vi "Configure Modulation (Phase).vi"(0 "VISA resource name":refnum<visa-resource-name>, 1 "Enable Phase Modulation (T: Enable)":bool=TRUE, 5 "Channel (0: Channel 1)":u16(ring) items=["Channel 1", "Channel 2"], 7 "PM Source (0: Internal)":u16(ring) items=["Internal", "External"], 9 "Modulation Waveform (0: Sine)":u16(ring) items=["Sine", "Square", "Triangle", "Ramp", "Down Ramp", "Noise", "User 1", "User 2", "User 3", "User 4", "Edit Memory"], 11 "error in (no error)":errorcluster, 12 "Modulation Frequency (100.00 Hz)":dbl=100.0 format="%#_6f", 13 "Peak Deviation (90 deg)":dbl=90.0 min=-180.0 max=180.0 format="%#.4f") -> (4 "VISA resource name out":refnum<visa-resource-name>, 15 "error out":errorcluster)   [LabVIEW 2013, in "Tektronix AFG 3000 Series.lvlib"]
doc: "Configures and enables phase modulation (PM). In PM, the phase of the carrier is varied by the peak deviation and the modulating waveform. \n\n<B>Note:</B>\n\nDefault measure for peak deviation is in degrees only. To change deviation unit to radians replace the DEG with RAD in the peak deviation command."
uses:
  Tektronix AFG 3000 Series.lvlib
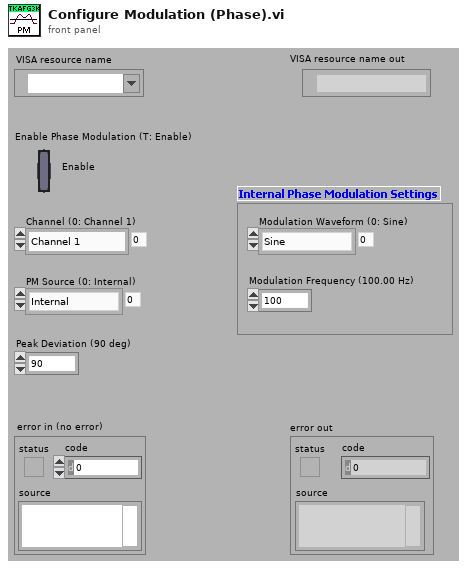
[diagram p1: front panel]
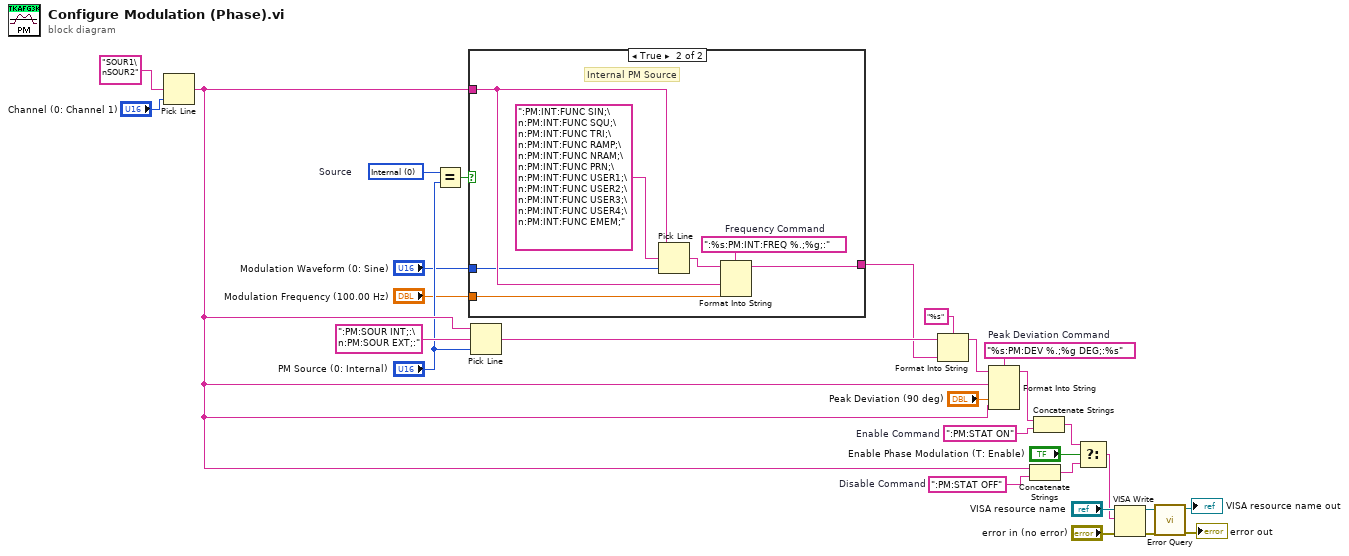
[diagram p0: block diagram]
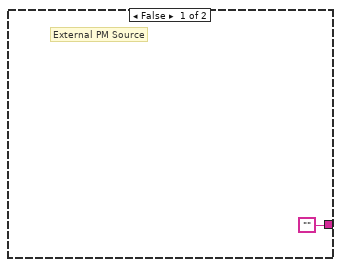
[diagram p2: hidden frame]
diagram:
  w20 = ":PM:STAT ON"  # Enable Command
  w22 = "%s:PM:DEV %.;%g DEG;:%s"  # Peak Deviation Command
  w9 = u16 0 items=["Internal", "External"]  # Source
  w17 = ":PM:STAT OFF"  # Disable Command
  n1 = Pick Line(multi-line string="SOUR1\nSOUR2" ("string (\"\")"), line index="Channel (0: Channel 1)") -> (output string=w11:string)  [unwired: 1 in]
  n2 = Equal?(x=w9, y="PM Source (0: Internal)") -> (x = y?=w8:bool)
  n3 = case shown="True" w8 {
    tunnel: ["" w33] -> w4
    tunnel: w11 -> [_ w32]
    tunnel: "Modulation Waveform (0: Sine)" -> [_ w31]
    tunnel: "Modulation Frequency (100.00 Hz)" -> [_ w30]
    frame False {
      # "External PM Source"
    }
    frame True {
      w34 = ":%s:PM:INT:FREQ %.;%g;:"  # Frequency Command
      # "Internal PM Source"
      n4 = Pick Line(string ("")=w32, multi-line string=":PM:INT:FUNC SIN;\n:PM:INT:FUNC SQU;\n:PM:INT:FUNC TRI;\n:PM:INT:FUNC RAMP;\n:PM:INT:FUNC NRAM;\n:PM:INT:FUNC PRN;\n:PM:INT:FUNC USER1;\n:PM:INT:FUNC USER2;\n:PM:INT:FUNC USER3;\n:PM:INT:FUNC USER4;\n:PM:INT:FUNC EMEM;", line index=w31) -> (output string=w35:string)
      n5 = Format Into String(format string=w34, initial string=w35, w32, w30) -> (resulting string=w33:string)  [unwired: 1 in, 1 out]
    }
  }
  n6 = Pick Line(string ("")=w11, multi-line string=":PM:SOUR INT;:\n:PM:SOUR EXT;:" ("Source Command"), line index="PM Source (0: Internal)") -> (output string=w5:string)
  n7 = Format Into String(format string="%s", initial string=w5, w4) -> (resulting string=w3:string)  [unwired: 1 in, 1 out]
  n8 = Format Into String(format string=w22, initial string=w3, w11, "Peak Deviation (90 deg)", w11) -> (resulting string=w21:string)  [unwired: 1 in, 1 out]
  n9 = Concatenate Strings(w11, w17) -> (w15:string)
  n10 = Concatenate Strings(w21, w20) -> (w14:string)
  n11 = Select(t=w14, s="Enable Phase Modulation (T: Enable)", f=w15) -> (s? t:f=w13:string)
  n12 = VISA Write(VISA resource name="VISA resource name", write buffer=w13, error in (no error)="error in (no error)") -> (VISA resource name out=w26:refnum<visa-resource-name>, error out=w25:errorcluster)  [unwired: 1 out]
  n13 = call "Error Query.vi"("error in (no error)"=w25, "VISA resource name"=w26) -> ("error out"=→"error out":errorcluster, "VISA resource name out"=→"VISA resource name out":refnum<visa-resource-name>)  [unwired: 6 in, 2 out]
